vi "4. NumericOps2.vi"() -> ()   [LabVIEW 2019]
panel:
  out "1/x":dbl
  out "x^2":dbl
  out "sqrt(x)":dbl
  out "x-1":dbl
  out "x+1":dbl
  in  "Num3":dbl
  out "floor(x/y)":dbl
  out "Remainder":dbl
  in  "Num2":dbl
  in  "Num1":dbl
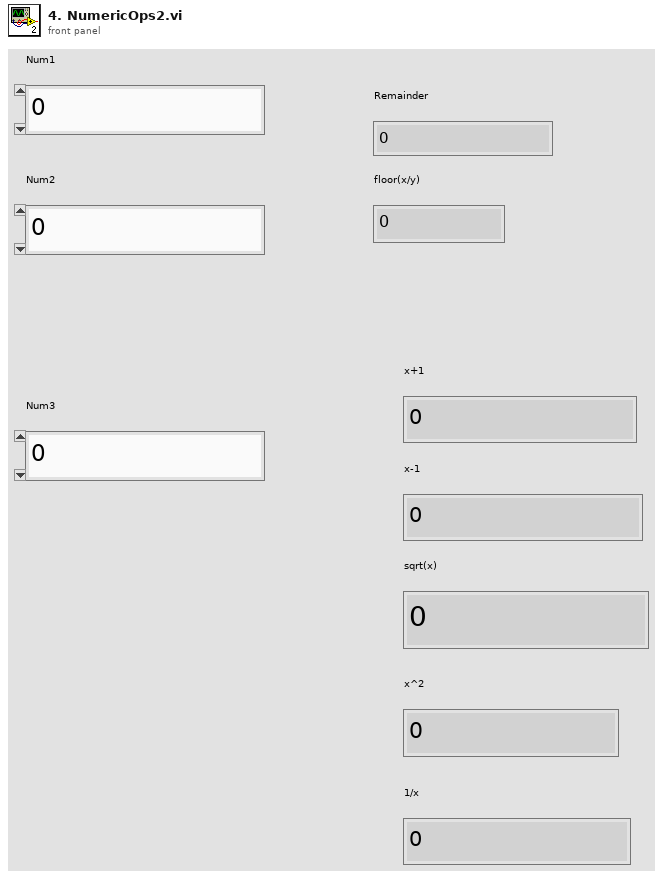
[diagram p1: front panel]
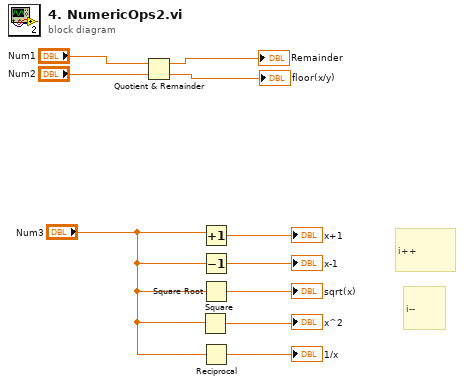
[diagram p0: block diagram]
diagram:
  # "i--"
  # "i++"
  n1 = Quotient & Remainder(x="Num1", y="Num2") -> (x-y*floor(x/y)=→"Remainder":dbl, floor(x/y)=→"floor(x/y)":dbl)
  n2 = Square(x="Num3") -> (x^2=→"x^2":dbl)
  n3 = Increment(x="Num3") -> (x+1=→"x+1":dbl)
  n4 = Decrement(x="Num3") -> (x-1=→"x-1":dbl)
  n5 = Square Root(x="Num3") -> (sqrt(x)=→"sqrt(x)":dbl)
  n6 = Reciprocal(x="Num3") -> (1/x=→"1/x":dbl)
